vi "Exponential Curve Fiting.vi"(4 "end":dbl=1.0 format="%0.2f", 5 "start":dbl format="%0.2f", 6 "Y":dbl[](array[numeric]), 7 "X":dbl[](array[numeric])) -> (0 "T Last":dbl, 1 "T First":dbl, 2 "XY Graph":cluster{"Ramp Pattern":dbl[], dbl[]}(graph))   [LabVIEW 2017]
uses:
  <vilib>/Analysis/1siggen.llb/Ramp Pattern by Samples.vi
  <vilib>/Analysis/NI_AALBase.lvlib
  <vilib>/Analysis/NI_AALPro.lvlib
panel:
  out "XY Graph 2":cluster{"Ramp Pattern":dbl[], dbl[]}(graph)
  in  "samples":i32=128
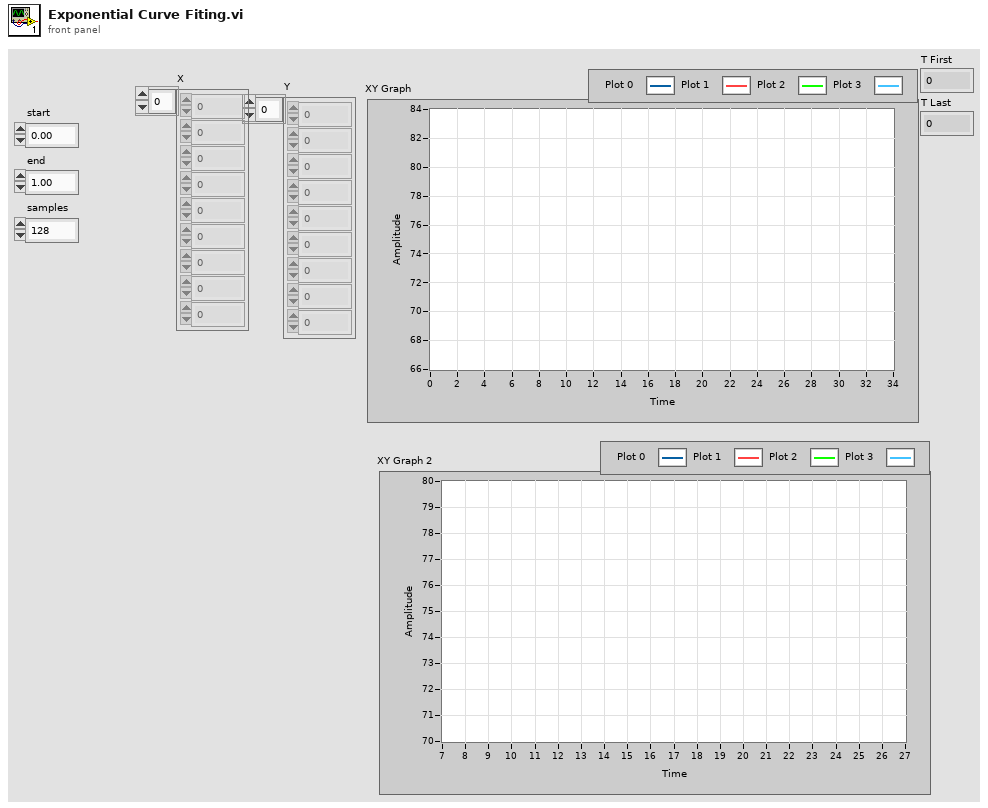
[diagram p1: front panel]
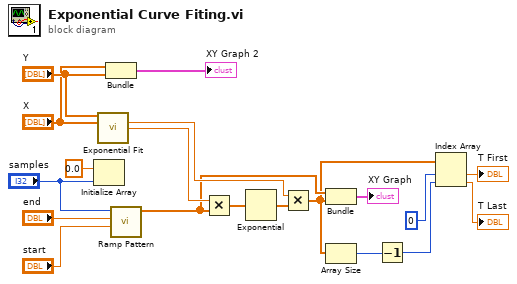
[diagram p0: block diagram]
diagram:
  n1 = Initialize Array(0.0 ("element"), "samples") -> ()  [unwired: 1 out]
  n2 = call <vilib>:"Exponential Fit.vi"("Y"="Y", "X"="X") -> ("amplitude"=w6:dbl, "damping"=w9:dbl)  [unwired: 8 in, 4 out]
  n3 = Bundle("X"="X", "Y"="Y") -> (→"XY Graph 2":cluster{"X":dbl[], "Y":dbl[]})  [unwired: 1 in]
  n4 = call-poly <vilib>:"Ramp Pattern.vi"("start"="start", "end"="end", "samples"="samples") -> ("Ramp Pattern"=w5:dbl[])  [unwired: 7 in, 1 out]
  n5 = Multiply(x=w9, y=w5) -> (x*y=w8:dbl[])
  n6 = Exponential(1:w8) -> (0:w7:dbl[])
  n7 = Multiply(x=w6, y=w7) -> (x*y=w3:dbl[])
  n8 = Bundle("Ramp Pattern"=w5, w3) -> (→"XY Graph":cluster{"Ramp Pattern":dbl[], dbl[]})  [unwired: 1 in]
  n9 = Array Size(array=w3) -> (size(s)=w15:i32)
  n10 = Decrement(x=w15) -> (x-1=w14:i32)
  n11 = Index Array(array=w3, index #1=0 ("index"), index #2=w14) -> (element #1=→"T First":dbl, element #2=→"T Last":dbl)
